vi "get channels.vi"(11 "Profibus Module configuration in":refnum<class "Profibus Module configuration.lvclass">) -> (2 "channels":refnum<class "TBM channel.lvclass">[](array[class]), 3 "Profibus Module configuration out":refnum<class "Profibus Module configuration.lvclass">)   [LabVIEW 2013, in "Profibus Module configuration.lvclass"]
uses:
  Profibus Module configuration.lvclass
  <vilib>/NI/Tag Bus Module Framework/channel/TBM channel.lvclass
  Profibus Module configuration.lvclass/Profibus Module configuration.ctl
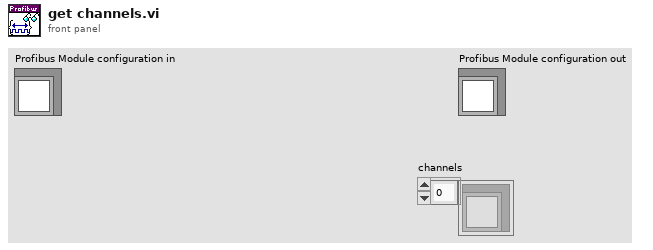
[diagram p1: front panel]
types:
  T1 = typedef "Profibus Module configuration.lvclass/slave diagnostic configuration.ctl" = cluster{"slave":i8, "report":bool, "channel":refnum<class "TBM channel.lvclass">, "error specs":T2[]}
  T2 = typedef "Profibus Module configuration.lvclass/error throw specification.ctl" = cluster{"byte":i32, "bit":i32, "inverted?":bool, "error":i32}
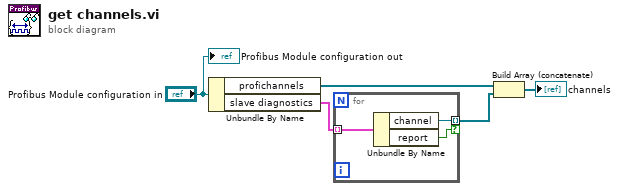
[diagram p0: block diagram]
diagram:
  n1 = Unbundle By Name("Profibus Module configuration in") -> ("profichannels"=w1:refnum<class "Profibus channel.lvclass">[], "slave diagnostics"=w4:T1[])
  n2 = for {
    tunnel: w4 -> [w8] mode=indexing
    tunnel: [w7] -> w3 mode=indexing if=w6
    n3 = Unbundle By Name(w8) -> ("channel"=w7:refnum<class "TBM channel.lvclass">, "report"=w6:bool)
  }
  n4 = Build Array (concatenate)(w1, w3) -> (→"channels":refnum<class "TBM channel.lvclass">[])
  "Profibus Module configuration out" <- "Profibus Module configuration in"
